vi "Run the cron command.vi"() -> ()   [LabVIEW 2017]
uses:
  System.Windows.Forms
  <vilib>/httpClient/LabVIEWHTTPClient.lvlib
panel:
  in  "WebView2":refnum<k24>(container)
  in  "WebBrowser":refnum<k24>(container)
  out "body":string
  out "standard output":string
  out "Error Out":errorcluster
  in  "Error In":errorcluster
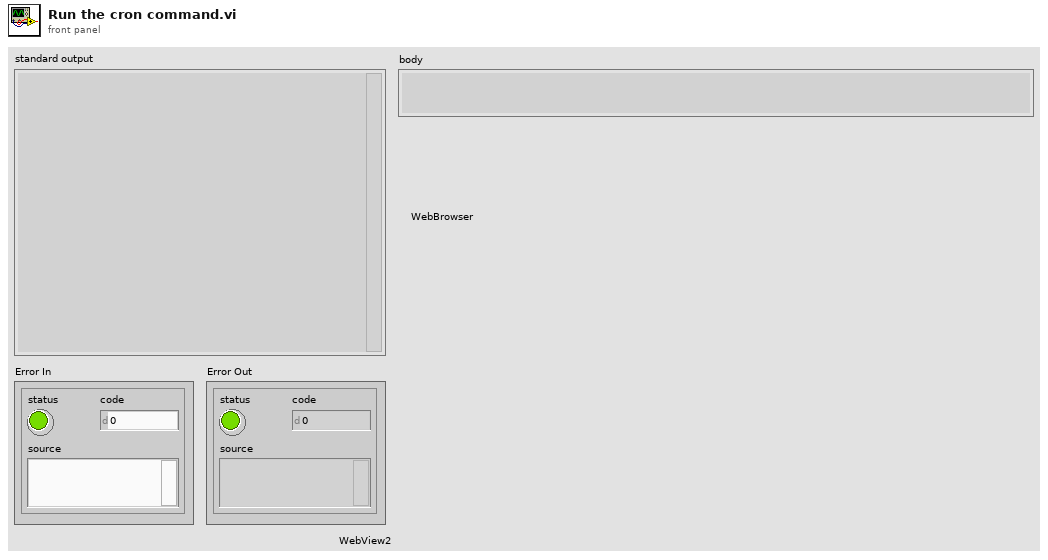
[diagram p1: front panel]
types:
  T1 = typedef "LabVIEWHTTPClient.lvlib/ClientHandle.ctl" = refnum<k1>
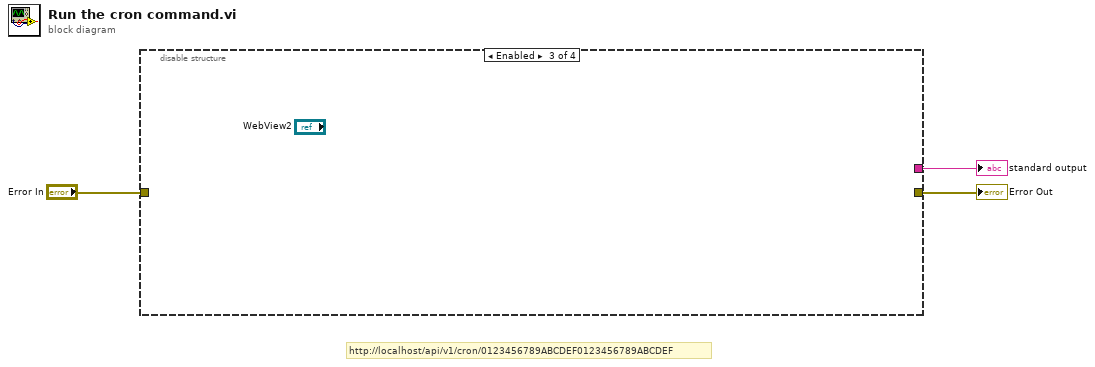
[diagram p0: block diagram]
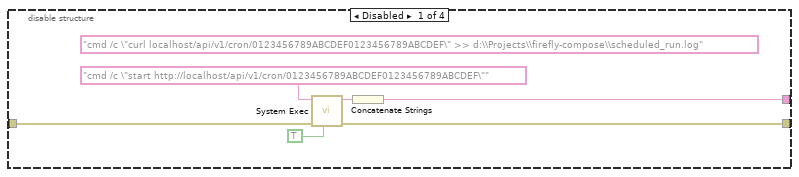
[diagram p2: hidden frame]
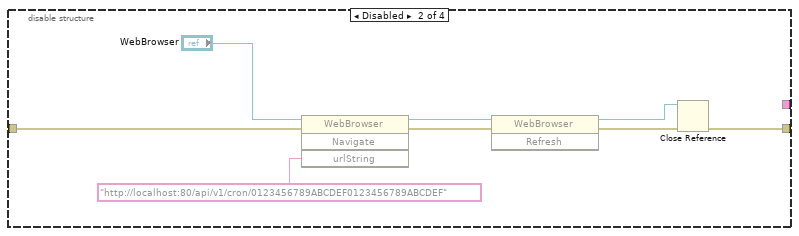
[diagram p3: hidden frame]
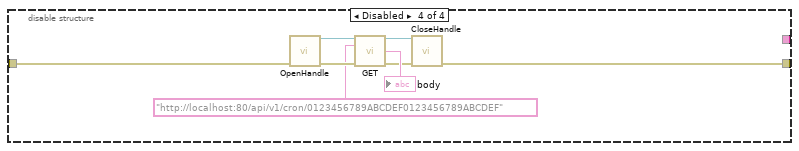
[diagram p4: hidden frame]
diagram:
  # "http://localhost/api/v1/cron/0123456789ABCDEF0123456789ABCDEF"
  n1 = disable-structure shown="Enabled" {
    disable-tunnel: "Error In" -> [w9 w15 _ w19]
    disable-tunnel: [w8 w14 _ w18] -> w2
    disable-tunnel: [w5 _ _ _] -> w1
    frame Disabled {
      (unwired) "cmd /c \"curl localhost/api/v1/cron/0123456789ABCDEF0123456789ABCDEF\" >> d:\\Projects\\firefly-compose\\scheduled_run.log"
      n2 = call <vilib>:"System Exec.vi"("run minimized? (F)"=TRUE, "error in (no error)"=w9, "command line"="cmd /c \"start http://localhost/api/v1/cron/0123456789ABCDEF0123456789ABCDEF\"") -> ("error out"=w8:errorcluster, "standard output"=w6:string)  [unwired: 5 in, 2 out]
      n3 = Concatenate Strings(w6) -> (w5:string)
    }
    frame Disabled {
      n4 = invoke class="WebBrowser" method="Navigate"(reference="WebBrowser", error in=w15, "urlString"="http://localhost:80/api/v1/cron/0123456789ABCDEF0123456789ABCDEF") -> (reference out=w13:refnum<k24>, error out=w11:errorcluster)  [unwired: 1 in, 2 out]
      n5 = invoke class="WebBrowser" method="Refresh"(reference=w13, error in=w11) -> (reference out=w12:refnum<k24>, error out=w10:errorcluster)  [unwired: 1 in, 1 out]
      n6 = Close Reference(reference=w12, error in (no error)=w10) -> (error out=w14:errorcluster)
    }
    frame Enabled {
    }
    frame Disabled {
      n7 = call <vilib>:"OpenHandle.vi"("error in (no error)"=w19) -> ("client handle out"=w21:T1, "error out"=w23:errorcluster)  [unwired: 13 in]
      n8 = call <vilib>:"GET.vi"("client handle"=w21, "url"="http://localhost:80/api/v1/cron/0123456789ABCDEF0123456789ABCDEF", "error in (no error)"=w23) -> ("client handle out"=w22:T1, "body"=→"body":string, "error out"=w24:errorcluster)  [unwired: 9 in, 1 out]
      n9 = call <vilib>:"CloseHandle.vi"("client handle"=w22, "error in (no error)"=w24) -> ("error out"=w18:errorcluster)  [unwired: 13 in]
    }
  }
  "Error Out" <- w2
  "standard output" <- w1
